vi "pt2waveform.vi"(4 "interp. oversampling factor":i32, 6 "interp method (nearest)":T1(ring)=enum."nearest", 7 "reset?":bool, 8 "history to keep (10k)":i32=10000 format="%.0p", 9 "history to display (1k)":i32=1000 format="%.0p", 10 "dt from last data point":dbl format="%.2p s", 11 "input data point":variant) -> (2 "waveform":waveform(dbl)(graph) caption="Waveform")   [LabVIEW 2015]
uses:
  <vilib>/Analysis/baseanly.llb/Mean (DBL).vi
  <vilib>/Analysis/1siggen.llb/Ramp Pattern by Samples.vi
  <vilib>/ptbypt/NI_PtbyPt.lvlib
  <vilib>/Analysis/NI_AALBase.lvlib
  <vilib>/gmath/NI_Gmath.lvlib
  <vilib>/Utility/Data Type/NI_Data Type.lvlib
panel:
  out "dt out":dbl format="%#_6p s"
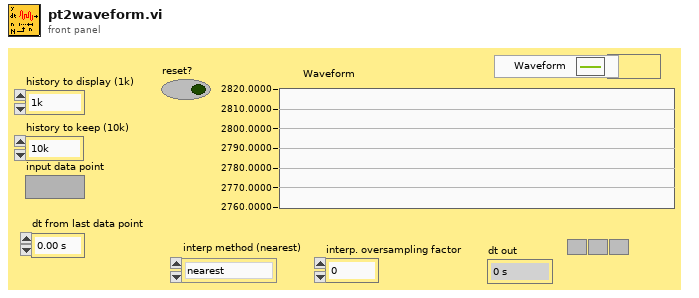
[diagram p1: front panel]
types:
  T1 = enum16{"none", "nearest", "linear", "spline", "cubic Hermite", "Lagrange"}
  T2 = typedef "LVNumericRepresentation.ctl" = enum32{"Extended Precision", "Double Precision", "Single Precision", "Long", "Word", "Byte", "Unsigned Long", "Unsigned Word", "Unsigned Byte", "Complex Extended", "Complex Double", "Complex Single", "Quad", "Unsigned Quad", "Fixed-Point"}
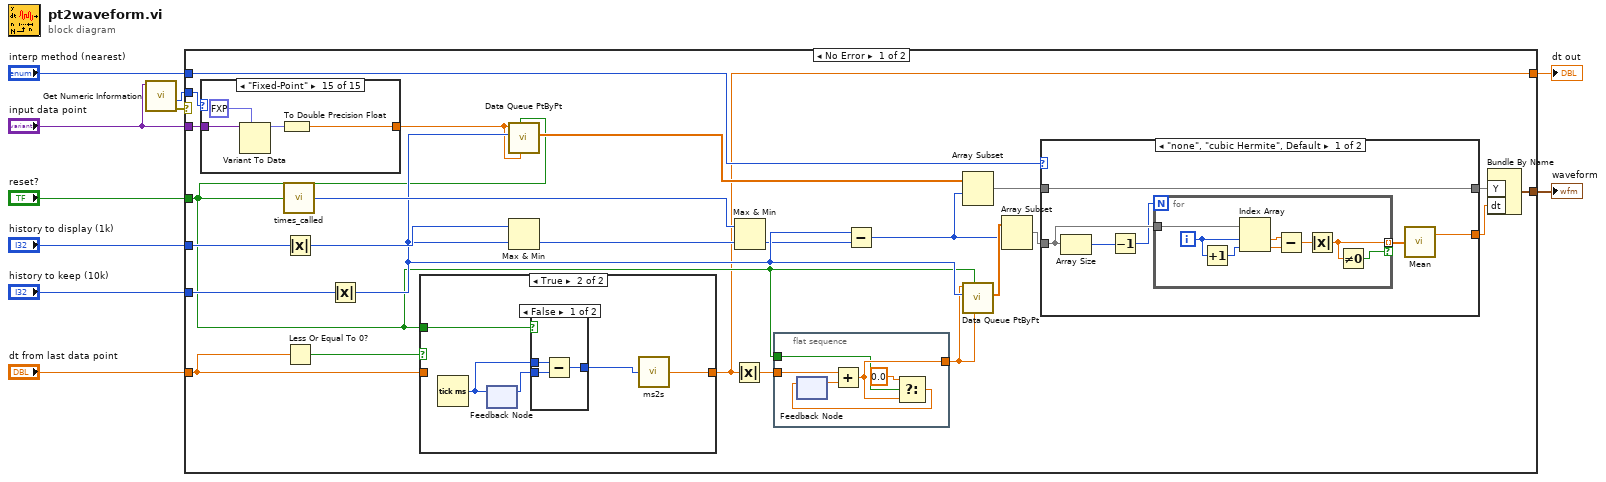
[diagram p0: block diagram]
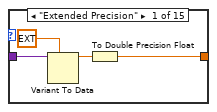
[diagram p2: hidden frame]
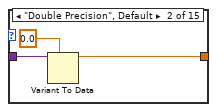
[diagram p3: hidden frame]
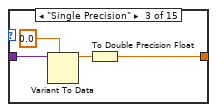
[diagram p4: hidden frame]
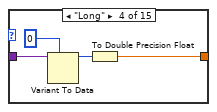
[diagram p5: hidden frame]
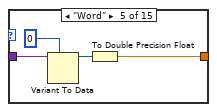
[diagram p6: hidden frame]
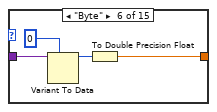
[diagram p7: hidden frame]
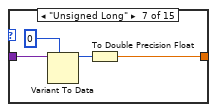
[diagram p8: hidden frame]
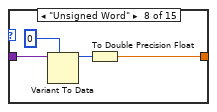
[diagram p9: hidden frame]
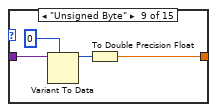
[diagram p10: hidden frame]
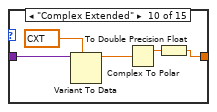
[diagram p11: hidden frame]
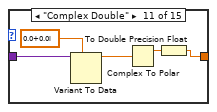
[diagram p12: hidden frame]
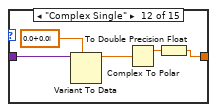
[diagram p13: hidden frame]
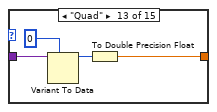
[diagram p14: hidden frame]
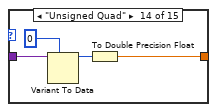
[diagram p15: hidden frame]
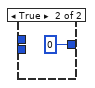
[diagram p17: hidden frame]
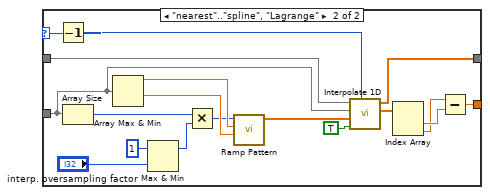
[diagram p18: hidden frame]
diagram:
  n1 = call <vilib>:"Get Numeric Information.vi"("Variant"="input data point") -> ("error out"=w3:errorcluster, "Representation"=w1:T2)  [unwired: 7 in, 2 out]
  n2 = case shown="No Error" w3 {
    tunnel: [w28 _] -> w10
    tunnel: "interp method (nearest)" -> [w27 _]
    tunnel: "history to display (1k)" -> [w24 _]
    tunnel: "history to keep (10k)" -> [w22 _]
    tunnel: "dt from last data point" -> [w16 w146]
    tunnel: "reset?" -> [w15 _]
    tunnel: [w14 w146] -> w4
    tunnel: "input data point" -> [w12 _]
    tunnel: w1 -> [w13 _]
    frame No Error {
      n3 = case shown="\"Fixed-Point\"" w13 {
        tunnel: w12 -> [w38 w42 w46 w50 w52 w56 w60 w64 w68 w74 w77 w82 w87 w91 w95]
        tunnel: [w36 w40 w43 w47 w51 w55 w59 w63 w67 w71 w76 w81 w86 w90 w94] -> w11
        frame "Extended Precision" {
          n4 = Variant To Data(type=ext 0.0, Variant=w38) -> (data=w37:ext)  [unwired: 1 in, 1 out]
          n5 = To Double Precision Float(number=w37) -> (double precision float=w36:dbl)
        }
        frame "Double Precision", Default {
          n6 = Variant To Data(type=0.0, Variant=w42) -> (data=w40:dbl)  [unwired: 1 in, 1 out]
        }
        frame "Single Precision" {
          n7 = Variant To Data(type=sgl 0.0, Variant=w46) -> (data=w44:sgl)  [unwired: 1 in, 1 out]
          n8 = To Double Precision Float(number=w44) -> (double precision float=w43:dbl)
        }
        frame "Long" {
          n9 = Variant To Data(type=0, Variant=w50) -> (data=w48:i32)  [unwired: 1 in, 1 out]
          n10 = To Double Precision Float(number=w48) -> (double precision float=w47:dbl)
        }
        frame "Word" {
          n11 = Variant To Data(type=i16 0, Variant=w52) -> (data=w53:i16)  [unwired: 1 in, 1 out]
          n12 = To Double Precision Float(number=w53) -> (double precision float=w51:dbl)
        }
        frame "Byte" {
          n13 = Variant To Data(type=i8 0, Variant=w56) -> (data=w57:i8)  [unwired: 1 in, 1 out]
          n14 = To Double Precision Float(number=w57) -> (double precision float=w55:dbl)
        }
        frame "Unsigned Long" {
          n15 = Variant To Data(type=u32 0, Variant=w60) -> (data=w61:u32)  [unwired: 1 in, 1 out]
          n16 = To Double Precision Float(number=w61) -> (double precision float=w59:dbl)
        }
        frame "Unsigned Word" {
          n17 = Variant To Data(type=u16 0, Variant=w64) -> (data=w65:u16)  [unwired: 1 in, 1 out]
          n18 = To Double Precision Float(number=w65) -> (double precision float=w63:dbl)
        }
        frame "Unsigned Byte" {
          n19 = Variant To Data(type=u8 0, Variant=w68) -> (data=w69:u8)  [unwired: 1 in, 1 out]
          n20 = To Double Precision Float(number=w69) -> (double precision float=w67:dbl)
        }
        frame "Complex Extended" {
          n21 = Variant To Data(type=cxt 0.0+0.0i, Variant=w74) -> (data=w73:cxt)  [unwired: 1 in, 1 out]
          n22 = Complex To Polar(r * e^(i*theta)=w73) -> (r=w72:ext)  [unwired: 1 out]
          n23 = To Double Precision Float(number=w72) -> (double precision float=w71:dbl)
        }
        frame "Complex Double" {
          n24 = Variant To Data(type=cdb 0.0+0.0i, Variant=w77) -> (data=w79:cdb)  [unwired: 1 in, 1 out]
          n25 = Complex To Polar(r * e^(i*theta)=w79) -> (r=w78:dbl)  [unwired: 1 out]
          n26 = To Double Precision Float(number=w78) -> (double precision float=w76:dbl)
        }
        frame "Complex Single" {
          n27 = Variant To Data(type=csg 0.0+0.0i, Variant=w82) -> (data=w84:csg)  [unwired: 1 in, 1 out]
          n28 = Complex To Polar(r * e^(i*theta)=w84) -> (r=w83:sgl)  [unwired: 1 out]
          n29 = To Double Precision Float(number=w83) -> (double precision float=w81:dbl)
        }
        frame "Quad" {
          n30 = Variant To Data(type=i64 0, Variant=w87) -> (data=w88:i64)  [unwired: 1 in, 1 out]
          n31 = To Double Precision Float(number=w88) -> (double precision float=w86:dbl)
        }
        frame "Unsigned Quad" {
          n32 = Variant To Data(type=u64 0, Variant=w91) -> (data=w92:u64)  [unwired: 1 in, 1 out]
          n33 = To Double Precision Float(number=w92) -> (double precision float=w90:dbl)
        }
        frame "Fixed-Point" {
          n34 = Variant To Data(type=fxp<+,1,1> 0.0, Variant=w95) -> (data=w96:fxp<+,1,1>)  [unwired: 1 in, 1 out]
          n35 = To Double Precision Float(number=w96) -> (double precision float=w94:dbl)
        }
      }
      n36 = call "times_called.vi"("reset?"=w15) -> ("times called"=w26:i32)  [unwired: 8 in]
      n37 = Absolute Value(x=w24) -> (abs(x)=w23:i32)
      n38 = Less Or Equal To 0?(x=w16) -> (x <= 0?=w17:bool)
      n39 = Absolute Value(x=w22) -> (abs(x)=w21:i32)
      n40 = case shown="True" w17 {
        tunnel: [w98 w99] -> w14
        tunnel: w16 -> [w98 _]
        tunnel: w15 -> [_ w103]
        frame False {
        }
        frame True {
          n41 = Tick Count (ms)() -> (millisecond timer value=w102:u32)
          n42 = feedback #1() -> (w101:u32)  [unwired: 1 in]
          n43 = feedback-in #1(w102) -> ()
          n44 = case shown="False" w103 {
            tunnel: [w106 u32 0] -> w100
            tunnel: w101 -> [w105 _]
            tunnel: w102 -> [w104 _]
            frame False {
              n45 = Subtract(x=w104, y=w105) -> (x-y=w106:u32)
            }
            frame True {
            }
          }
          n46 = call "ms2s.vi"("ms"=w100) -> ("s"=w99:dbl)  [unwired: 4 in]
        }
      }
      n47 = call <vilib>:"Data Queue PtByPt.vi"("initial queue element"=w11, "initialize"=w15, "sample length"=w21, "input data point"=w11) -> ("Current Queue"=w33:dbl[])  [unwired: 3 in, 4 out]
      n48 = Max & Min(x=w23, y=w21) -> (min(x,y)=w25:i32)  [unwired: 1 out]
      n49 = Absolute Value(x=w14) -> (abs(x)=w19:dbl)
      n50 = Max & Min(x=w26, y=w25) -> (min(x,y)=w18:i32)  [unwired: 1 out]
      n51 = flat-sequence {
        tunnel: [w111] -> w20
        tunnel: w15 -> [w110]
        tunnel: w19 -> [w108]
        frame #0 {
          n52 = feedback #2() -> (w113:dbl)  [unwired: 1 in]
          n53 = Add(x=w108, y=w113) -> (x+y=w111:dbl)
          n54 = Select(t=0.0, s=w110, f=w111) -> (s? t:f=w109:dbl)
          n55 = feedback-in #2(w109) -> ()
        }
      }
      n56 = Subtract(x=w21, y=w18) -> (x-y=w29:i32)
      n57 = Array Subset(array=w33, index=w29) -> (w32:dbl[])  [unwired: 1 in]
      n58 = call <vilib>:"Data Queue PtByPt.vi"("initial queue element"=w20, "initialize"=w15, "sample length"=w21, "input data point"=w20) -> ("Current Queue"=w31:dbl[])  [unwired: 3 in, 4 out]
      n59 = Array Subset(array=w31, index=w29) -> (w30:dbl[])  [unwired: 1 in]
      n60 = case shown="\"none\", \"cubic Hermite\", Default" w27 {
        selector: w27 -> [_ w135]
        tunnel: [w117 w142] -> w35
        tunnel: [w119 w139] -> w34
        tunnel: w32 -> [w119 w137]
        tunnel: w30 -> [w116 w136]
        frame "none", "cubic Hermite", Default {
          n61 = Array Size(array=w116) -> (size(s)=w115:i32)
          n62 = Decrement(x=w115) -> (x-1=w114:i32)
          n63 = for {
            N: w114 -> [_]
            tunnel: w116 -> [w126]
            tunnel: [w120] -> w118 mode=indexing if=w121
            i -> [w124]
            n64 = Increment(x=w124) -> (x+1=w123:i32)
            n65 = Index Array(array=w126, index #1=w124, index #2=w123) -> (element #1=w125:dbl, element #2=w122:dbl)
            n66 = Subtract(x=w125, y=w122) -> (x-y=w127:dbl)
            n67 = Absolute Value(x=w127) -> (abs(x)=w120:dbl)
            n68 = Not Equal To 0?(x=w120) -> (x != 0?=w121:bool)
          }
          n69 = call-poly <vilib>:"Mean.vi"("X"=w118) -> ("mean"=w117:dbl)  [unwired: 1 out]
        }
        frame "nearest".."spline", "Lagrange" {
          n70 = Decrement(x=w135) -> (x-1=w128:T1)
          n71 = Array Size(array=w136) -> (size(s)=w133:i32)
          n72 = Array Max & Min(array=w136) -> (max value=w145:dbl, min value=w144:dbl)  [unwired: 2 out]
          n73 = Max & Min(x=1, y="interp. oversampling factor") -> (max(x,y)=w129:i32)  [unwired: 1 out]
          n74 = Multiply(x=w133, y=w129) -> (x*y=w132:i32)
          n75 = call-poly <vilib>:"Ramp Pattern.vi"("start"=w144, "end"=w145, "samples"=w132) -> ("Ramp Pattern"=w143:dbl[])  [unwired: 7 in, 1 out]
          n76 = call <vilib>:"Interpolate 1D.vi"("method"=w128, "X is monotonic"=TRUE, "xi"=w143, "X"=w136, "Y"=w137) -> ("xi used"=w138:dbl[], "yi"=w139:dbl[])  [unwired: 4 in, 1 out]
          n77 = Index Array(array=w138) -> (element #1=w141:dbl, element #2=w140:dbl)  [unwired: 2 in]
          n78 = Subtract(x=w140, y=w141) -> (x-y=w142:dbl)
        }
      }
      n79 = Bundle By Name("Y"=w34, "dt"=w35) -> (w28:waveform(dbl))  [unwired: 1 out]
    }
    frame Error {
    }
  }
  "waveform" <- w10
  "dt out" <- w4
